vi "HapticSTM_Feedblackless_testdata.vi"() -> ()   [LabVIEW 2017]
uses:
  <userlib>/HapticSTM/Feedbackless - Testdata/HapticSTM_Feedblackless_testdata Folder/HapticSTM.lvlib
  <userlib>/HapticSTM/Feedbackless - Testdata/HapticSTM_Feedblackless_testdata Folder/GlobalClicksHeight.vi
  <vilib>/ptbypt/NI_PtbyPt.lvlib
  <vilib>/Utility/file.llb/Read Delimited Spreadsheet (DBL).vi
  <vilib>/Analysis/3filter.llb/Filter Passband Type.ctl
  <vilib>/Analysis/NI_AALBase.lvlib
panel:
  in  "Force Mode":u16(ring) items=["Stacked Logs", "Simple Log", "Linear"]
  out "Button":bool
  out "Zpos":cluster{dbl, "Y":dbl, i16}(graph)
  out "Filtered Current":dbl
  in  "Reset Clicks":bool
  out "Scaled Force and Current":cluster{dbl, "Filtered x":dbl, dbl}(graph)
  in  "Maximum (pA)":dbl=9000.0
  in  "Setpoint (pA)":dbl=100.0
  out "PLANE HEIGHT":dbl
  out "Current":dbl
  out "Origin Y":dbl
  out "Origin X":dbl
  out "Output Z":dbl
  in  "Rough adjust":dbl
  out "Nano Z":dbl
  out "Width":dbl
  out "VY":dbl
  out "VZ":dbl
  out "VX":dbl
  in  "Drag":dbl=1.0
  in  "STOP":bool
  in  "START":bool
  out "Fy":dbl
  out "Fz":dbl
  out "phi":dbl
  out "psi":dbl
  out "Fx":dbl
  out "theta":dbl
  out "x":dbl
  out "y":dbl
  out "z":dbl
  in  "Fine adjust":dbl=3.5
  out "Clicks":dbl
  out "Height":dbl
  # "Sample Window"
  # "Position"
  # "Sensitivity"
  # "Force"
  # "STM I/O"
  # "Angles"
  # "Current"
  # "Velocity"
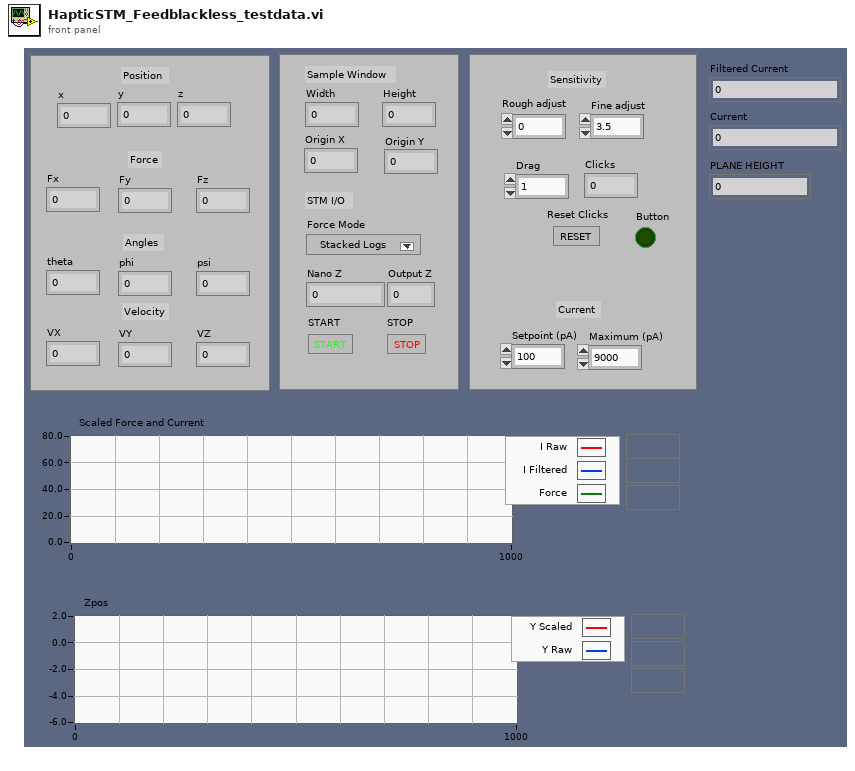
[diagram p1: front panel]
types:
  T1 = typedef "NI_AALBase.lvlib/Filter Passband Type.ctl" = enum32{"Lowpass", "Highpass", "Bandpass", "Bandstop"}
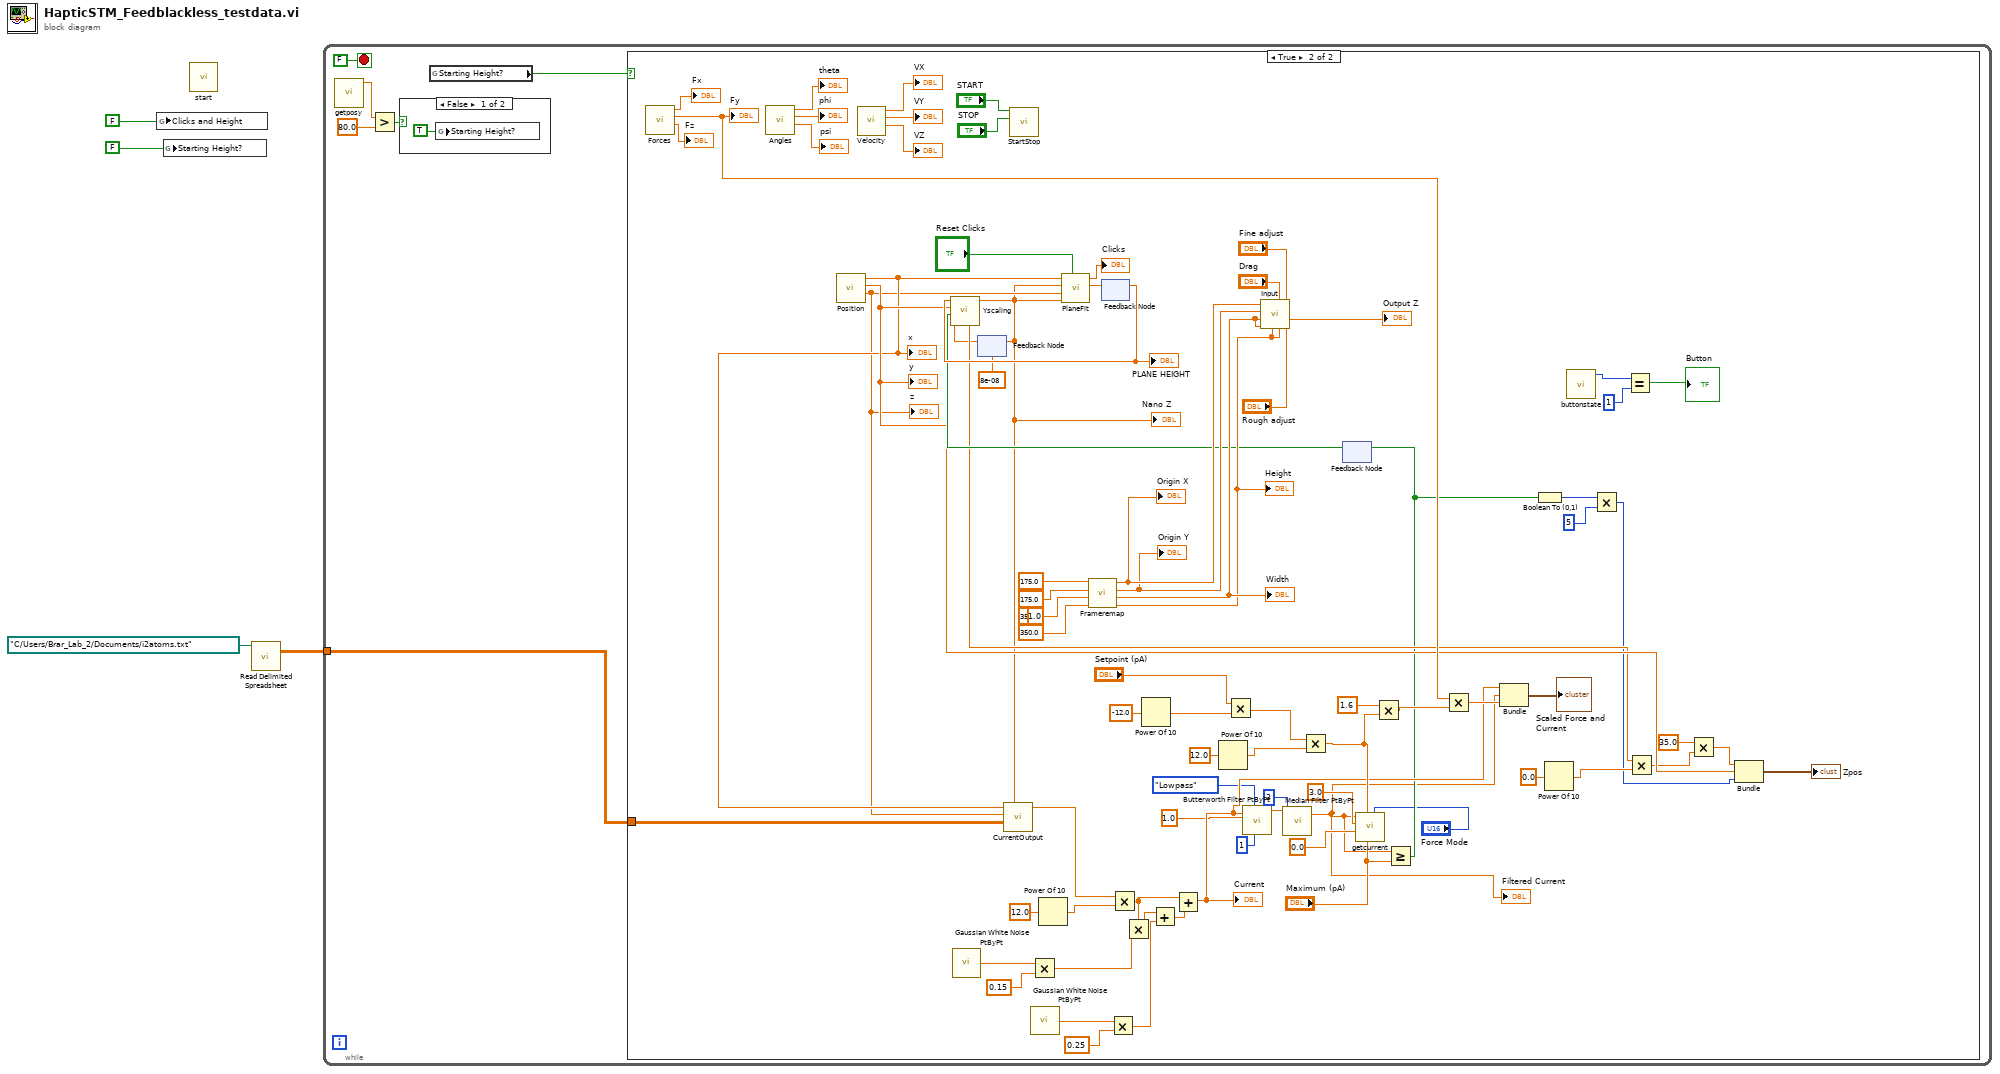
[diagram p0: block diagram]
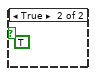
[diagram p2: hidden frame]
diagram:
  n1 = global write "GlobalClicksHeight.vi" "Clicks and Height"(FALSE ("Clicks and Height")) -> ()
  n2 = global write "GlobalClicksHeight.vi" "Starting Height?"(FALSE ("Clicks and Height")) -> ()
  n3 = call <userlib>:"start.vi"() -> ()  [unwired: 11 in, 1 out]
  n4 = call-poly <vilib>:"Read Delimited Spreadsheet.vi"("file path (dialog if empty)"=path "C:/Users/Brar_Lab_2/Documents/i2atoms.txt") -> ("all rows"=w4:dbl[][])  [unwired: 9 in, 5 out]
  n5 = while {
    tunnel: w4 -> [w10]
    stop <- FALSE stop-if-true
    n6 = call <userlib>:"getposy.vi"() -> ("function return"=w9:dbl)  [unwired: 11 in]
    n7 = Greater?(x=w9, y=80.0) -> (0:w7:bool)
    n8 = case shown="False" w7 {
      frame False {
        n9 = global write "GlobalClicksHeight.vi" "Starting Height?"(TRUE ("Starting Height?")) -> ()
      }
      frame True {
        (unwired) TRUE ("Clicks and Height")
      }
    }
    n10 = global read "GlobalClicksHeight.vi" "Starting Height?"() -> (w6:bool)
    n11 = case shown="True" w6 {
      tunnel: w10 -> [_ w13]
      frame False {
      }
      frame True {
        (unwired) 1.0 ("FO X")
        n12 = call <userlib>:"Forces.vi"() -> ("Fz"=→"Fz":dbl, "Fy"=w56:dbl, "Fx"=→"Fx":dbl)  [unwired: 9 in]
        "Fy" <- w56
        n13 = call <userlib>:"Angles.vi"() -> ("psi"=→"psi":dbl, "phi"=→"phi":dbl, "theta"=→"theta":dbl)  [unwired: 9 in]
        n14 = call <userlib>:"Position.vi"() -> ("Z"=w14:dbl, "Y"=w38:dbl, "X"=w15:dbl)  [unwired: 9 in]
        "x" <- w15
        "y" <- w38
        "z" <- w14
        n15 = call <userlib>:"Velocity.vi"() -> ("VZ"=→"VZ":dbl, "VY"=→"VY":dbl, "VX"=→"VX":dbl)  [unwired: 9 in]
        n16 = call <vilib>:"Gaussian White Noise PtByPt.vi"() -> ("Gaussian white noise"=w55:dbl)  [unwired: 3 in]
        n17 = feedback #1(8e-08 ("y scaled")) -> (w19:dbl)
        n18 = call <userlib>:"StartStop.vi"("STOP"="STOP", "START"="START") -> ()  [unwired: 10 in]
        n19 = Multiply(x=w55, y=0.15) -> (x*y=w53:dbl)
        n20 = call <vilib>:"Gaussian White Noise PtByPt.vi"() -> ("Gaussian white noise"=w50:dbl)  [unwired: 3 in]
        n21 = Power Of 10(x=12.0) -> (10^x=w74:dbl)
        n22 = call <userlib>:"Frameremap.vi"("FH"=350.0 ("FO X"), "FW"=350.0 ("FO X"), "FO Z"=175.0 ("FO X"), "FO X"=175.0) -> ("FH"=w81:dbl, "FW"=w82:dbl, "Z Origin"=w66:dbl, "X Origin"=w67:dbl)  [unwired: 4 in]
        "Height" <- w81
        "Width" <- w82
        "Origin X" <- w67
        "Origin Y" <- w66
        n23 = feedback #2() -> (w68:dbl)  [unwired: 1 in]
        "PLANE HEIGHT" <- w68
        n24 = Multiply(x=w50, y=0.25) -> (x*y=w46:dbl)
        n25 = Power Of 10(x=-12.0) -> (10^x=w63:dbl)
        n26 = Power Of 10(x=12.0) -> (10^x=w65:dbl)
        n27 = Multiply(x="Setpoint (pA)", y=w63) -> (x*y=w61:dbl)
        n28 = call <userlib>:"Input.vi"("Current * 10^input"="Rough adjust", "Sensitivity"="Fine adjust", "Scopez"=w81, "Drag"="Drag", "FH"=w81, "FW"=w82, "Scopex"=w82, "Z origin"=w66, "X origin"=w67) -> ("Scaled Current"=→"Output Z":dbl)  [unwired: 2 in]
        n29 = Multiply(x=w61, y=w65) -> (x*y=w43:dbl)
        n30 = feedback #3() -> (w59:bool)  [unwired: 1 in]
        n31 = call <userlib>:"Yscaling.vi"("Nano Z Read"=w19, "Current Maxed?"=w59, "Y"=w38, "Plane Height"=w68) -> ("y scaled"=w12:dbl, "Testoutput"=w34:dbl)  [unwired: 6 in]
        "Nano Z" <- w12
        n32 = feedback-in #1(w12) -> ()
        n33 = call <userlib>:"CurrentOutput.vi"("y scaled"=w12, "array"=w13, "Z Input"=w14, "X Input"=w15) -> ("Current Out"=w16:dbl)  [unwired: 7 in]
        n34 = call <userlib>:"PlaneFit.vi"("Reset Clicks"="Reset Clicks", "Y PEN"=w12, "Z"=w14, "Nano Z"=w12, "X"=w15) -> ("Plane Height (m)"=w77:dbl, "Clicks"=→"Clicks":dbl)  [unwired: 5 in]
        n35 = feedback-in #2(w77) -> ()
        n36 = Multiply(x=w16, y=w74) -> (x*y=w52:dbl)
        n37 = Multiply(x=w52, y=w53) -> (x*y=w47:dbl)
        n38 = Add(x=w47, y=w46) -> (x+y=w48:dbl)
        n39 = Add(x=w52, y=w48) -> (x+y=w30:dbl)
        "Current" <- w30
        n40 = call <vilib>:"Butterworth Filter PtByPt.vi"("order"=1, "filter type"=Filter_Passband_Type."Lowpass", "sampling freq: fs"=1.0, "x"=w30) -> ("Filtered x"=w22:dbl)  [unwired: 5 in, 1 out]
        n41 = call <vilib>:"Median Filter PtByPt.vi"("rank"=3, "x"=w22) -> ("Filtered x"=w21:dbl)  [unwired: 2 in, 1 out]
        "Filtered Current" <- w21
        n42 = call <userlib>:"getcurrent.vi"("forcemode"="Force Mode", "maxcurrentin"="Maximum (pA)", "setpoint"=w43, "minforcey"=0.0, "maxforcey"=3.0, "currentin"=w21) -> ()  [unwired: 6 in]
        n43 = Multiply(x=1.6 ("y"), y=w43) -> (x*y=w44:dbl)
        n44 = Greater Or Equal?(x=w21, y="Maximum (pA)") -> (x >= y?=w27:bool)
        n45 = feedback-in #3(w27) -> ()
        n46 = Multiply(x=w56, y=w44) -> (x*y=w51:dbl)
        n47 = Bundle(w30, "Filtered x"=w21, w51) -> (→"Scaled Force and Current":cluster{dbl, "Filtered x":dbl, dbl})  [unwired: 1 in]
        n48 = Boolean To (0,1)(Boolean=w27) -> (0, 1=w26:i16)
        n49 = Power Of 10(x=0.0) -> (10^x=w41:dbl)
        n50 = call <userlib>:"buttonstate.vi"() -> ("function return"=w33:i32)  [unwired: 11 in]
        n51 = Multiply(x=w26, y=i16 5) -> (x*y=w24:i16)
        n52 = Equal?(x=w33, y=1) -> (x = y?=→"Button":bool)
        n53 = Multiply(x=w34, y=w41) -> (x*y=w36:dbl)
        n54 = Multiply(x=35.0, y=w36) -> (x*y=w37:dbl)
        n55 = Bundle(w37, "Y"=w38, w24) -> (→"Zpos":cluster{dbl, "Y":dbl, i16})  [unwired: 1 in]
      }
    }
  }
